vi "test_SC.vi"() -> ()   [LabVIEW 2015]
uses:
  <vilib>/DAQmx/write.llb/DAQmx Write (Digital Bool 1Line 1Point).vi
  <vilib>/DAQmx/create/channels.llb/DAQmx Create Channel (DO-Digital Output).vi
  <vilib>/DAQmx/miscellaneous.llb/DAQmx Fill In Error Info.vi
panel:
  out "Waveform Graph":dbl[](graph)
  out "temps d'acqu ms":u32=4148
  in  "Number of scans":i32=1
  in  "stop":bool
  in  "Start":bool
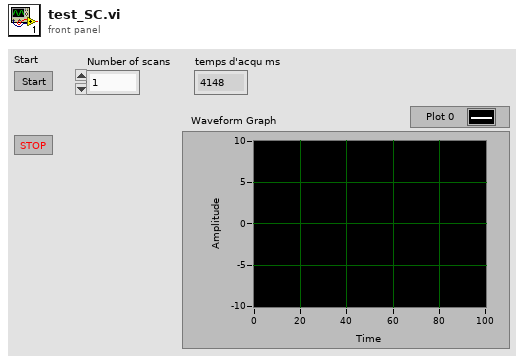
[diagram p1: front panel]
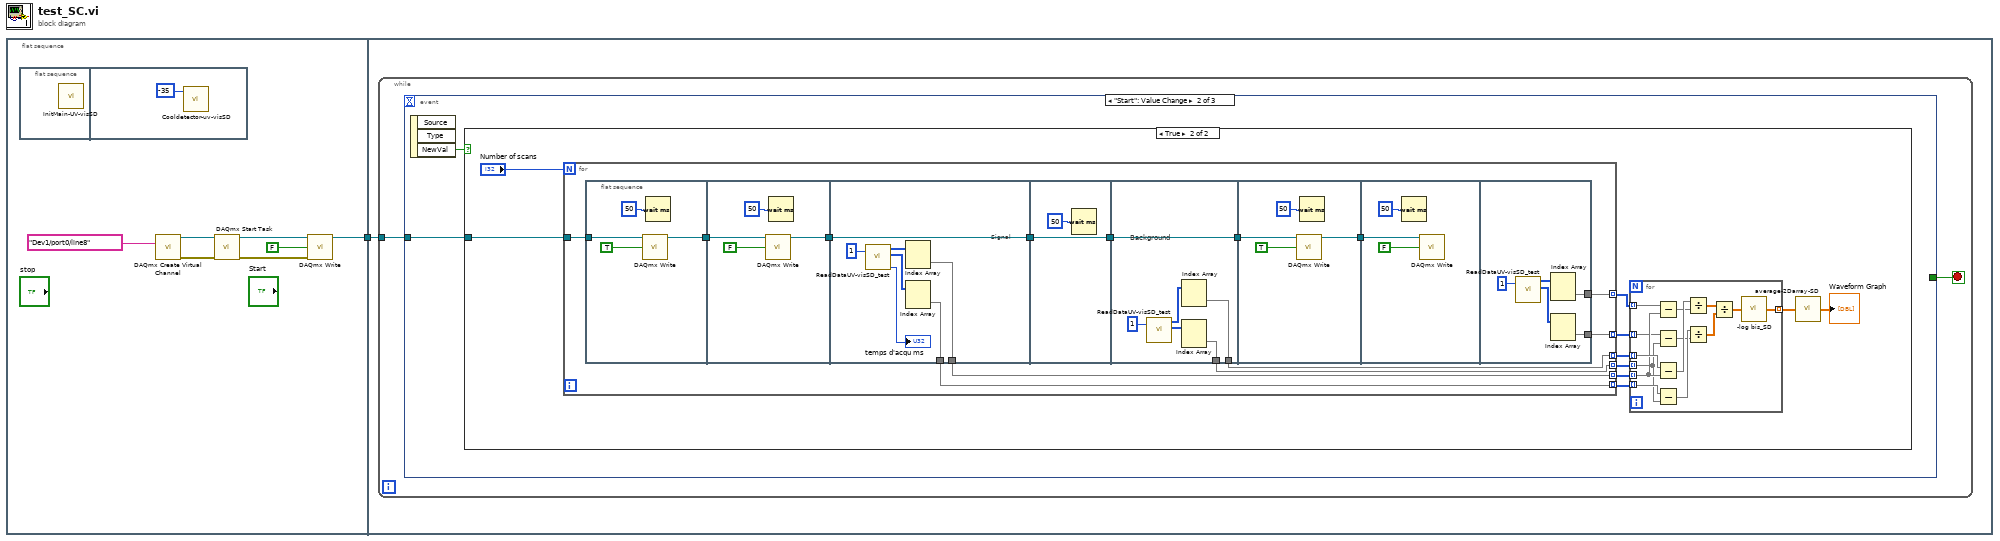
[diagram p0: block diagram]
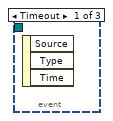
[diagram p2: hidden frame]
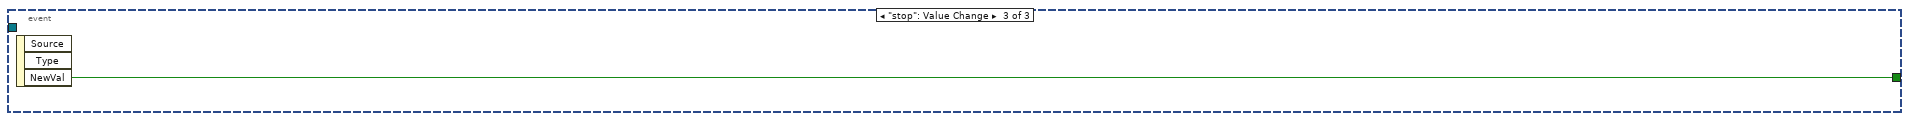
[diagram p4: hidden frame]
diagram:
  n1 = flat-sequence {
    tunnel: [w3] -> w1
    tunnel: w1 -> [w10]
    frame #0 {
      n2 = flat-sequence {
        frame #0 {
          n3 = call "InitMain-UV-visSD.vi"() -> ()  [unwired: 1 out]
        }
        frame #1 {
          n4 = call "Cooldetector-uv-visSD.vi"("temp set"=-35) -> ()  [unwired: 2 in, 2 out]
        }
      }
      n5 = call-poly <vilib>:"DAQmx Create Virtual Channel.vi"("lines"=tag "Dev1/port0/line8" ("Lines")) -> ("task out"=w7:refnum<k21>, "error out"=w6:errorcluster)  [unwired: 13 in]
      n6 = call <vilib>:"DAQmx Start Task.vi"("task/channels in"=w7, "error in"=w6) -> ("task out"=w8:refnum<k21>, "error out"=w5:errorcluster)  [unwired: 12 in]
      n7 = call-poly <vilib>:"DAQmx Write.vi"("task/channels in"=w8, "data"=FALSE, "error in"=w5) -> ("task out"=w3:refnum<k21>)  [unwired: 10 in, 2 out]
    }
    frame #1 {
      n8 = while {
        tunnel: w10 -> [w11]
        stop <- w12 stop-if-true
        n9 = event shown="[1] \"Start\": Value Change" {
          selector: _ -> [_ _ _]
          dyn-events: _ -> [_ _ _]
          timeout: _ -> [_ _ _]
          tunnel: [_ _ w87] -> w12
          tunnel: w11 -> [_ w14 _]
          event Timeout {
            n10 = event-data() -> ()  [unwired: 1 in, 3 out]
          }
          event "Start": Value Change {
            n11 = event-data() -> ("NewVal"=w13:bool)  [unwired: 1 in, 2 out]
            n12 = case shown="True" w13 {
              tunnel: w14 -> [_ w24]
              frame False {
              }
              frame True {
                n13 = for {
                  N: "Number of scans" -> [_]
                  tunnel: w24 -> [w50]
                  tunnel: [w44] -> w22 mode=indexing
                  tunnel: [w43] -> w17 mode=indexing
                  tunnel: [w42] -> w21 mode=indexing
                  tunnel: [w41] -> w16 mode=indexing
                  tunnel: [w40] -> w20 mode=indexing
                  tunnel: [w39] -> w15 mode=indexing
                  n14 = flat-sequence {
                    tunnel: w50 -> [w54]
                    tunnel: [w52] -> w51
                    tunnel: w51 -> [w59]
                    tunnel: [w56] -> w46
                    tunnel: [w64] -> w47
                    tunnel: w46 -> [w64]
                    tunnel: [w62] -> w44
                    tunnel: [w60] -> w43
                    tunnel: [w67] -> w48
                    tunnel: w47 -> [w67]
                    tunnel: [w73] -> w49
                    tunnel: w48 -> [w73]
                    tunnel: [w71] -> w42
                    tunnel: [w69] -> w41
                    tunnel: w49 -> [w76]
                    tunnel: [w75] -> w45
                    tunnel: w45 -> [w79]
                    tunnel: [w84] -> w40
                    tunnel: [w82] -> w39
                    frame #0 {
                      n15 = call-poly <vilib>:"DAQmx Write.vi"("task/channels in"=w54, "data"=TRUE) -> ("task out"=w52:refnum<k21>)  [unwired: 11 in, 2 out]
                      n16 = Wait (ms)(milliseconds to wait=u32 50) -> ()  [unwired: 1 out]
                    }
                    frame #1 {
                      n17 = call-poly <vilib>:"DAQmx Write.vi"("task/channels in"=w59, "data"=FALSE) -> ("task out"=w56:refnum<k21>)  [unwired: 11 in, 2 out]
                      n18 = Wait (ms)(milliseconds to wait=u32 50) -> ()  [unwired: 1 out]
                    }
                    frame #2 {
                      # "Signal"
                      n19 = call "ReadDataUV-visSD_test.vi"("Nombre de aq"=1) -> ("Channel I"=w63:i32[][], "Channel II"=w61:i32[][], "temps d'acqu ms"=→"temps d'acqu ms":u32)  [unwired: 1 in, 1 out]
                      n20 = Index Array(array=w63) -> (element=w62:i32[])  [unwired: 2 in]
                      n21 = Index Array(array=w61) -> (element=w60:i32[])  [unwired: 2 in]
                    }
                    frame #3 {
                      n22 = Wait (ms)(milliseconds to wait=u32 50) -> ()  [unwired: 1 out]
                    }
                    frame #4 {
                      # "Background"
                      n23 = call "ReadDataUV-visSD_test.vi"("Nombre de aq"=1) -> ("Channel I"=w72:i32[][], "Channel II"=w70:i32[][])  [unwired: 1 in, 2 out]
                      n24 = Index Array(array=w72) -> (element=w71:i32[])  [unwired: 2 in]
                      n25 = Index Array(array=w70) -> (element=w69:i32[])  [unwired: 2 in]
                    }
                    frame #5 {
                      n26 = call-poly <vilib>:"DAQmx Write.vi"("task/channels in"=w76, "data"=TRUE) -> ("task out"=w75:refnum<k21>)  [unwired: 11 in, 2 out]
                      n27 = Wait (ms)(milliseconds to wait=u32 50) -> ()  [unwired: 1 out]
                    }
                    frame #6 {
                      n28 = Wait (ms)(milliseconds to wait=u32 50) -> ()  [unwired: 1 out]
                      n29 = call-poly <vilib>:"DAQmx Write.vi"("task/channels in"=w79, "data"=FALSE) -> ()  [unwired: 11 in, 3 out]
                    }
                    frame #7 {
                      n30 = call "ReadDataUV-visSD_test.vi"("Nombre de aq"=1) -> ("Channel I"=w85:i32[][], "Channel II"=w83:i32[][])  [unwired: 1 in, 2 out]
                      n31 = Index Array(array=w85) -> (element=w84:i32[])  [unwired: 2 in]
                      n32 = Index Array(array=w83) -> (element=w82:i32[])  [unwired: 2 in]
                    }
                  }
                }
                n33 = for {
                  tunnel: w22 -> [w37] mode=indexing
                  tunnel: w21 -> [w38] mode=indexing
                  tunnel: w20 -> [w36] mode=indexing
                  tunnel: [w30] -> w19 mode=indexing
                  tunnel: w17 -> [w29] mode=indexing
                  tunnel: w16 -> [w28] mode=indexing
                  tunnel: w15 -> [w27] mode=indexing
                  n34 = Subtract(x=w36, y=w37) -> (x-y=w34:i32[])
                  n35 = Subtract(x=w27, y=w28) -> (x-y=w25:i32[])
                  n36 = Subtract(x=w38, y=w37) -> (x-y=w35:i32[])
                  n37 = Subtract(x=w29, y=w28) -> (x-y=w26:i32[])
                  n38 = Divide(x=w35, y=w34) -> (x/y=w33:dbl[])
                  n39 = Divide(x=w26, y=w25) -> (x/y=w32:dbl[])
                  n40 = Divide(x=w33, y=w32) -> (x/y=w31:dbl[])
                  n41 = call "-log bis_SD.vi"("Transmission"=w31) -> ("-log(x)=log(1/x)"=w30:dbl[])
                }
                n42 = call "average-2Darray-SD.vi"("2D array"=w19) -> ("out array"=→"Waveform Graph":dbl[])
              }
            }
          }
          event "stop": Value Change {
            n43 = event-data() -> ("NewVal"=w87:bool)  [unwired: 1 in, 2 out]
          }
        }
      }
    }
  }
